vi "Finish.vi"   [LabVIEW 2019]
doc: "This VIcloses device references, sends final commands to the network tables and the joysticks, and terminates all command and control loops."
uses:
  refnums.vi
  <vilib>/Rock Robotics/WPI/Utilities/WPI_GetSetVariantRefNum.vi
types:
  T1 = typedef "WPI_PotentiometerDevRef.ctl" = cluster{"DevStatus":errorcluster, "Analog Channel":T2, "Invert Output":bool}
  T2 = typedef "FPGA_AIChannel.ctl" = enum8{"AI 0", "AI 1", "AI 2", "AI 3", "AI MXP 0", "AI MXP 1", "AI MXP 2", "AI MXP 3", "Invalid"}
  T3 = typedef "WPI_MotorControlDeviceRef.ctl" = cluster{"DeviceStatus":errorcluster, "Type":T4, "PWM":cluster{"PWM Channel":T5, "DeadBand":T6}, "CAN":cluster{"Device Number":u8, "SetOutput VI Ref":variant, "GetOutput VI Ref":variant, "Enable VI Ref":variant, "Disable VI Ref":variant, "Data":variant}, "Invert":bool, "DIO PWM":cluster{"PWM \"Enable\" Channel":T5, "DIOChannel":T7, "PWM Rate":dbl}}
  T4 = typedef "WPI_MotorControlType.ctl" = enum16{"PWM", "CAN", "DIO PWM"}
  T5 = typedef "FPGA_DIOPWMChannel.ctl" = enum8{"PWM 0", "PWM 1", "PWM 2", "PWM 3", "PWM 4", "PWM 5", "PWM 6", "PWM 7", "PWM 8", "PWM 9", "PWM MXP 0", "PWM MXP 1", "PWM MXP 2", "PWM MXP 3", "PWM MXP 4", "PWM MXP 5", "PWM MXP 6", "PWM MXP 7", "PWM MXP 8", "PWM MXP 9", "Invalid"}
  T6 = typedef "WPI_PWMDeadband.ctl" = cluster{"Name":string, "maxPositivePwm":i32, "minPositivePwm":i32, "centerPwm":i32, "maxNegativePwm":i32, "minNegativePwm":i32, "angularRange":u16}
  T7 = typedef "FPGA_DIOChannel.ctl" = enum8{"DIO 0", "DIO 1", "DIO 2", "DIO 3", "DIO 4", "DIO 5", "DIO 6", "DIO 7", "DIO 8", "DIO 9", "DIO MXP 0", "DIO MXP 1", "DIO MXP 2", "DIO MXP 3", "DIO MXP 4", "DIO MXP 5", "DIO MXP 6", "DIO MXP 7", "DIO MXP 8", "DIO MXP 9", "DIO MXP 10", "DIO MXP 11", "DIO MXP 12", "DIO MXP 13", "DIO MXP 14", "DIO MXP 15", "SPI Port CS1", "SPI Port CS2", "SPI Port CS3", "SPI Port MISO", "SPI Port MOSI", "Invalid"}
  T8 = typedef "WPI_SolenoidDevRef.ctl" = cluster{"DevStatus":errorcluster, "Pneumatics Control Module":u8, "Forward Solenoid Channel":T9, "Reverse Solenoid Channel":T9}
  T9 = typedef "WPI_SolenoidChannel.ctl" = enum8{"Solenoid 0", "Solenoid 1", "Solenoid 2", "Solenoid 3", "Solenoid 4", "Solenoid 5", "Solenoid 6", "Solenoid 7", "Invalid"}
  T10 = typedef "WPI_AnalogChannelDevRef.ctl" = cluster{"DevStatus":errorcluster, "Analog Channel":T2}
  T11 = typedef "WPI_CounterDevRef.ctl" = cluster{"DevStatus":errorcluster, "CntIndex":T12}
  T12 = typedef "FPGA_CounterCtrSystemIndex.ctl" = enum8{"Ctr 0", "Ctr 1", "Ctr 2", "Ctr 3", "Ctr 4", "Ctr 5", "Ctr 6", "Ctr 7", "Invalid"}
  T13 = typedef "WPI_JoystickDevRef.ctl" = cluster{"Device":T14}
  T14 = typedef "WPI_JoystickDeviceEnum.ctl" = enum16{"USB 0", "USB 1", "USB 2", "USB 3", "USB 4", "USB 5"}
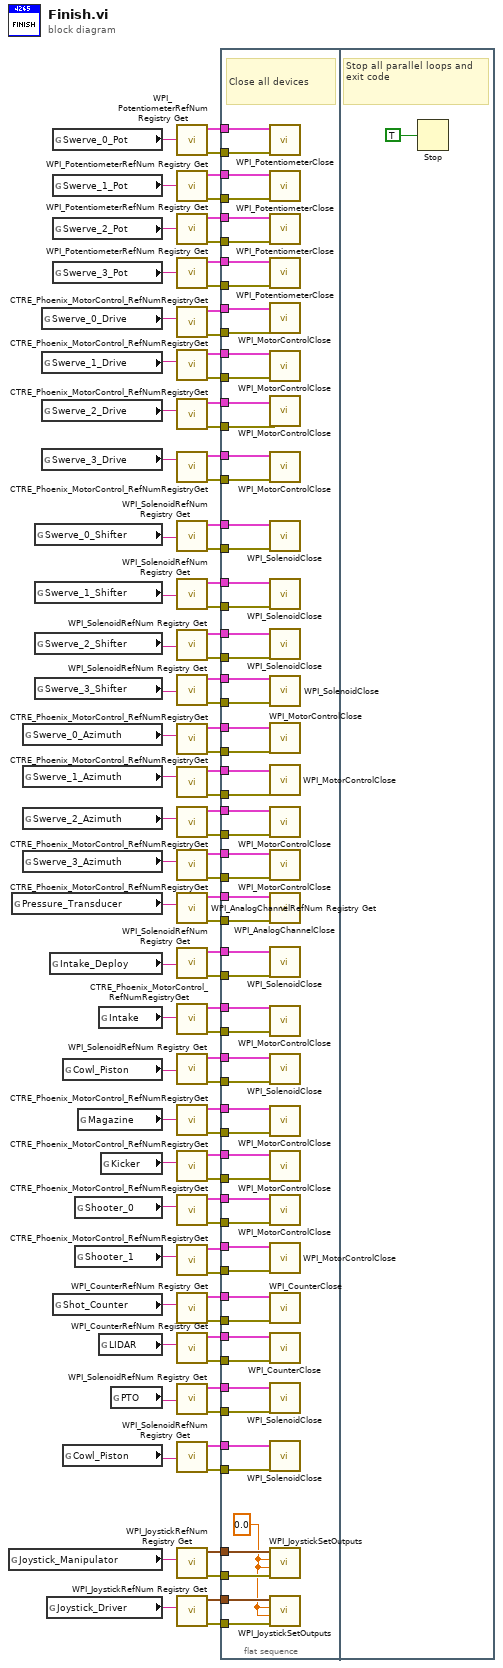
[diagram p0: block diagram]
diagram:
  n1 = global read "refnums.vi" "Joystick_Manipulator"() -> (w72:string)
  n2 = global read "refnums.vi" "Pressure_Transducer"() -> (w78:string)
  n3 = global read "refnums.vi" "Swerve_0_Azimuth"() -> (w48:string)
  n4 = global read "refnums.vi" "Swerve_1_Azimuth"() -> (w47:string)
  n5 = global read "refnums.vi" "Swerve_2_Azimuth"() -> (w46:string)
  n6 = global read "refnums.vi" "Swerve_3_Azimuth"() -> (w45:string)
  n7 = global read "refnums.vi" "Swerve_0_Shifter"() -> (w31:string)
  n8 = global read "refnums.vi" "Swerve_1_Shifter"() -> (w32:string)
  n9 = global read "refnums.vi" "Swerve_2_Shifter"() -> (w33:string)
  n10 = global read "refnums.vi" "Swerve_3_Shifter"() -> (w60:string)
  n11 = global read "refnums.vi" "Swerve_0_Drive"() -> (w57:string)
  n12 = global read "refnums.vi" "Swerve_1_Drive"() -> (w54:string)
  n13 = global read "refnums.vi" "Swerve_2_Drive"() -> (w52:string)
  n14 = global read "refnums.vi" "Swerve_3_Drive"() -> (w63:string)
  n15 = global read "refnums.vi" "Joystick_Driver"() -> (w67:string)
  n16 = global read "refnums.vi" "Intake_Deploy"() -> (w75:string)
  n17 = global read "refnums.vi" "Swerve_0_Pot"() -> (w90:string)
  n18 = global read "refnums.vi" "Swerve_1_Pot"() -> (w88:string)
  n19 = global read "refnums.vi" "Swerve_2_Pot"() -> (w87:string)
  n20 = global read "refnums.vi" "Swerve_3_Pot"() -> (w86:string)
  n21 = global read "refnums.vi" "Shot_Counter"() -> (w24:string)
  n22 = global read "refnums.vi" "Cowl_Piston"() -> (w23:string)
  n23 = global read "refnums.vi" "Cowl_Piston"() -> (w6:string)
  n24 = global read "refnums.vi" "Shooter_0"() -> (w12:string)
  n25 = global read "refnums.vi" "Shooter_1"() -> (w15:string)
  n26 = global read "refnums.vi" "Magazine"() -> (w20:string)
  n27 = global read "refnums.vi" "Intake"() -> (w36:string)
  n28 = global read "refnums.vi" "LIDAR"() -> (w66:string)
  n29 = global read "refnums.vi" "Kicker"() -> (w9:string)
  n30 = global read "refnums.vi" "PTO"() -> (w5:string)
  n31 = call <vilib>:"WPI_PotentiometerRefNum Registry Get.vi"("refnum name"=w90) -> ("error out"=w82:errorcluster, "PotDevRef"=w89:T1)  [unwired: 9 in]
  n32 = call <vilib>:"WPI_PotentiometerRefNum Registry Get.vi"("refnum name"=w88) -> ("error out"=w81:errorcluster, "PotDevRef"=w85:T1)  [unwired: 9 in]
  n33 = call <vilib>:"WPI_PotentiometerRefNum Registry Get.vi"("refnum name"=w87) -> ("error out"=w80:errorcluster, "PotDevRef"=w84:T1)  [unwired: 9 in]
  n34 = call <vilib>:"WPI_PotentiometerRefNum Registry Get.vi"("refnum name"=w86) -> ("error out"=w79:errorcluster, "PotDevRef"=w83:T1)  [unwired: 9 in]
  n35 = call <vilib>:"CTRE_Phoenix_MotorControl_RefNumRegistryGet.vi"("refnum name"=w57) -> ("error out"=w55:errorcluster, "PhoenixMotorControlDevRef"=w56:T3)  [unwired: 9 in]
  n36 = call <vilib>:"CTRE_Phoenix_MotorControl_RefNumRegistryGet.vi"("refnum name"=w54) -> ("error out"=w49:errorcluster, "PhoenixMotorControlDevRef"=w53:T3)  [unwired: 9 in]
  n37 = call <vilib>:"CTRE_Phoenix_MotorControl_RefNumRegistryGet.vi"("refnum name"=w52) -> ("error out"=w50:errorcluster, "PhoenixMotorControlDevRef"=w51:T3)  [unwired: 9 in]
  n38 = call <vilib>:"CTRE_Phoenix_MotorControl_RefNumRegistryGet.vi"("refnum name"=w63) -> ("error out"=w61:errorcluster, "PhoenixMotorControlDevRef"=w62:T3)  [unwired: 9 in]
  n39 = call <vilib>:"WPI_SolenoidRefNum Registry Get.vi"("refnum name"=w31) -> ("error out"=w29:errorcluster, "SolenoidDevRef"=w30:T8)  [unwired: 9 in]
  n40 = call <vilib>:"WPI_SolenoidRefNum Registry Get.vi"("refnum name"=w32) -> ("error out"=w27:errorcluster, "SolenoidDevRef"=w28:T8)  [unwired: 9 in]
  n41 = call <vilib>:"WPI_SolenoidRefNum Registry Get.vi"("refnum name"=w33) -> ("error out"=w25:errorcluster, "SolenoidDevRef"=w26:T8)  [unwired: 9 in]
  n42 = call <vilib>:"WPI_SolenoidRefNum Registry Get.vi"("refnum name"=w60) -> ("error out"=w58:errorcluster, "SolenoidDevRef"=w59:T8)  [unwired: 9 in]
  n43 = call <vilib>:"CTRE_Phoenix_MotorControl_RefNumRegistryGet.vi"("refnum name"=w48) -> ("error out"=w40:errorcluster, "PhoenixMotorControlDevRef"=w44:T3)  [unwired: 9 in]
  n44 = call <vilib>:"CTRE_Phoenix_MotorControl_RefNumRegistryGet.vi"("refnum name"=w47) -> ("error out"=w39:errorcluster, "PhoenixMotorControlDevRef"=w43:T3)  [unwired: 9 in]
  n45 = call <vilib>:"CTRE_Phoenix_MotorControl_RefNumRegistryGet.vi"("refnum name"=w46) -> ("error out"=w38:errorcluster, "PhoenixMotorControlDevRef"=w42:T3)  [unwired: 9 in]
  n46 = call <vilib>:"CTRE_Phoenix_MotorControl_RefNumRegistryGet.vi"("refnum name"=w45) -> ("error out"=w37:errorcluster, "PhoenixMotorControlDevRef"=w41:T3)  [unwired: 9 in]
  n47 = call <vilib>:"WPI_AnalogChannelRefNum Registry Get.vi"("refnum name"=w78) -> ("error out"=w76:errorcluster, "AIDeviceRef"=w77:T10)  [unwired: 9 in]
  n48 = call <vilib>:"WPI_SolenoidRefNum Registry Get.vi"("refnum name"=w75) -> ("error out"=w73:errorcluster, "SolenoidDevRef"=w74:T8)  [unwired: 9 in]
  n49 = call <vilib>:"CTRE_Phoenix_MotorControl_RefNumRegistryGet.vi"("refnum name"=w36) -> ("error out"=w34:errorcluster, "PhoenixMotorControlDevRef"=w35:T3)  [unwired: 9 in]
  n50 = call <vilib>:"WPI_SolenoidRefNum Registry Get.vi"("refnum name"=w23) -> ("error out"=w21:errorcluster, "SolenoidDevRef"=w22:T8)  [unwired: 9 in]
  n51 = call <vilib>:"CTRE_Phoenix_MotorControl_RefNumRegistryGet.vi"("refnum name"=w20) -> ("error out"=w18:errorcluster, "PhoenixMotorControlDevRef"=w19:T3)  [unwired: 9 in]
  n52 = call <vilib>:"CTRE_Phoenix_MotorControl_RefNumRegistryGet.vi"("refnum name"=w9) -> ("error out"=w7:errorcluster, "PhoenixMotorControlDevRef"=w8:T3)  [unwired: 9 in]
  n53 = call <vilib>:"CTRE_Phoenix_MotorControl_RefNumRegistryGet.vi"("refnum name"=w12) -> ("error out"=w10:errorcluster, "PhoenixMotorControlDevRef"=w11:T3)  [unwired: 9 in]
  n54 = call <vilib>:"CTRE_Phoenix_MotorControl_RefNumRegistryGet.vi"("refnum name"=w15) -> ("error out"=w13:errorcluster, "PhoenixMotorControlDevRef"=w14:T3)  [unwired: 9 in]
  n55 = call <vilib>:"WPI_CounterRefNum Registry Get.vi"("refnum name"=w24) -> ("error out"=w16:errorcluster, "CounterDevRef"=w17:T11)  [unwired: 9 in]
  n56 = call <vilib>:"WPI_CounterRefNum Registry Get.vi"("refnum name"=w66) -> ("error out"=w64:errorcluster, "CounterDevRef"=w65:T11)  [unwired: 9 in]
  n57 = call <vilib>:"WPI_SolenoidRefNum Registry Get.vi"("refnum name"=w5) -> ("error out"=w3:errorcluster, "SolenoidDevRef"=w4:T8)  [unwired: 9 in]
  n58 = call <vilib>:"WPI_SolenoidRefNum Registry Get.vi"("refnum name"=w6) -> ("error out"=w1:errorcluster, "SolenoidDevRef"=w2:T8)  [unwired: 9 in]
  n59 = call <vilib>:"WPI_JoystickRefNum Registry Get.vi"("refnum name"=w72) -> ("error out"=w70:errorcluster, "JoystickDevRef"=w71:T13)  [unwired: 9 in]
  n60 = call <vilib>:"WPI_JoystickRefNum Registry Get.vi"("refnum name"=w67) -> ("error out"=w68:errorcluster, "JoystickDevRef"=w69:T13)  [unwired: 9 in]
  n61 = flat-sequence {
    tunnel: w89 -> [w151]
    tunnel: w85 -> [w150]
    tunnel: w84 -> [w149]
    tunnel: w83 -> [w148]
    tunnel: w56 -> [w147]
    tunnel: w53 -> [w146]
    tunnel: w82 -> [w145]
    tunnel: w81 -> [w144]
    tunnel: w80 -> [w143]
    tunnel: w79 -> [w142]
    tunnel: w55 -> [w141]
    tunnel: w77 -> [w140]
    tunnel: w76 -> [w139]
    tunnel: w74 -> [w138]
    tunnel: w73 -> [w137]
    tunnel: w71 -> [w136]
    tunnel: w70 -> [w135]
    tunnel: w69 -> [w134]
    tunnel: w68 -> [w133]
    tunnel: w65 -> [w131]
    tunnel: w64 -> [w130]
    tunnel: w62 -> [w129]
    tunnel: w61 -> [w128]
    tunnel: w59 -> [w127]
    tunnel: w58 -> [w126]
    tunnel: w51 -> [w125]
    tunnel: w50 -> [w124]
    tunnel: w49 -> [w123]
    tunnel: w44 -> [w122]
    tunnel: w43 -> [w121]
    tunnel: w42 -> [w120]
    tunnel: w41 -> [w119]
    tunnel: w40 -> [w118]
    tunnel: w39 -> [w117]
    tunnel: w38 -> [w116]
    tunnel: w37 -> [w115]
    tunnel: w35 -> [w114]
    tunnel: w34 -> [w113]
    tunnel: w30 -> [w112]
    tunnel: w29 -> [w111]
    tunnel: w28 -> [w110]
    tunnel: w27 -> [w109]
    tunnel: w26 -> [w108]
    tunnel: w25 -> [w107]
    tunnel: w22 -> [w106]
    tunnel: w21 -> [w105]
    tunnel: w19 -> [w104]
    tunnel: w18 -> [w103]
    tunnel: w17 -> [w102]
    tunnel: w16 -> [w101]
    tunnel: w13 -> [w100]
    tunnel: w14 -> [w99]
    tunnel: w11 -> [w98]
    tunnel: w10 -> [w97]
    tunnel: w8 -> [w96]
    tunnel: w7 -> [w95]
    tunnel: w4 -> [w94]
    tunnel: w3 -> [w93]
    tunnel: w2 -> [w92]
    tunnel: w1 -> [w91]
    frame #0 {
      w132 = sgl 0.0 ("Left Rumble")
      # "Close all devices"
      n62 = call <vilib>:"WPI_PotentiometerClose.vi"("error in"=w145, "PotDevRef"=w151) -> ()  [unwired: 9 in, 1 out]
      n63 = call <vilib>:"WPI_PotentiometerClose.vi"("error in"=w144, "PotDevRef"=w150) -> ()  [unwired: 9 in, 1 out]
      n64 = call <vilib>:"WPI_PotentiometerClose.vi"("error in"=w143, "PotDevRef"=w149) -> ()  [unwired: 9 in, 1 out]
      n65 = call <vilib>:"WPI_PotentiometerClose.vi"("error in"=w142, "PotDevRef"=w148) -> ()  [unwired: 9 in, 1 out]
      n66 = call <vilib>:"WPI_MotorControlClose.vi"("error in"=w141, "MotorControlDevRef"=w147) -> ()  [unwired: 9 in, 1 out]
      n67 = call <vilib>:"WPI_MotorControlClose.vi"("error in"=w123, "MotorControlDevRef"=w146) -> ()  [unwired: 9 in, 1 out]
      n68 = call <vilib>:"WPI_MotorControlClose.vi"("error in"=w124, "MotorControlDevRef"=w125) -> ()  [unwired: 9 in, 1 out]
      n69 = call <vilib>:"WPI_MotorControlClose.vi"("error in"=w128, "MotorControlDevRef"=w129) -> ()  [unwired: 9 in, 1 out]
      n70 = call <vilib>:"WPI_SolenoidClose.vi"("error in (no error)"=w111, "SolenoidDevRef"=w112) -> ()  [unwired: 9 in, 1 out]
      n71 = call <vilib>:"WPI_SolenoidClose.vi"("error in (no error)"=w109, "SolenoidDevRef"=w110) -> ()  [unwired: 9 in, 1 out]
      n72 = call <vilib>:"WPI_SolenoidClose.vi"("error in (no error)"=w107, "SolenoidDevRef"=w108) -> ()  [unwired: 9 in, 1 out]
      n73 = call <vilib>:"WPI_SolenoidClose.vi"("error in (no error)"=w126, "SolenoidDevRef"=w127) -> ()  [unwired: 9 in, 1 out]
      n74 = call <vilib>:"WPI_MotorControlClose.vi"("error in"=w118, "MotorControlDevRef"=w122) -> ()  [unwired: 9 in, 1 out]
      n75 = call <vilib>:"WPI_MotorControlClose.vi"("error in"=w117, "MotorControlDevRef"=w121) -> ()  [unwired: 9 in, 1 out]
      n76 = call <vilib>:"WPI_MotorControlClose.vi"("error in"=w116, "MotorControlDevRef"=w120) -> ()  [unwired: 9 in, 1 out]
      n77 = call <vilib>:"WPI_MotorControlClose.vi"("error in"=w115, "MotorControlDevRef"=w119) -> ()  [unwired: 9 in, 1 out]
      n78 = call <vilib>:"WPI_AnalogChannelClose.vi"("error in (no error)"=w139, "AIDeviceRef"=w140) -> ()  [unwired: 9 in, 1 out]
      n79 = call <vilib>:"WPI_SolenoidClose.vi"("error in (no error)"=w137, "SolenoidDevRef"=w138) -> ()  [unwired: 9 in, 1 out]
      n80 = call <vilib>:"WPI_MotorControlClose.vi"("error in"=w113, "MotorControlDevRef"=w114) -> ()  [unwired: 9 in, 1 out]
      n81 = call <vilib>:"WPI_SolenoidClose.vi"("error in (no error)"=w105, "SolenoidDevRef"=w106) -> ()  [unwired: 9 in, 1 out]
      n82 = call <vilib>:"WPI_MotorControlClose.vi"("error in"=w103, "MotorControlDevRef"=w104) -> ()  [unwired: 9 in, 1 out]
      n83 = call <vilib>:"WPI_MotorControlClose.vi"("error in"=w95, "MotorControlDevRef"=w96) -> ()  [unwired: 9 in, 1 out]
      n84 = call <vilib>:"WPI_MotorControlClose.vi"("error in"=w97, "MotorControlDevRef"=w98) -> ()  [unwired: 9 in, 1 out]
      n85 = call <vilib>:"WPI_MotorControlClose.vi"("error in"=w100, "MotorControlDevRef"=w99) -> ()  [unwired: 9 in, 1 out]
      n86 = call <vilib>:"WPI_CounterClose.vi"("error in (no error)"=w101, "CounterDevRef"=w102) -> ()  [unwired: 9 in, 1 out]
      n87 = call <vilib>:"WPI_CounterClose.vi"("error in (no error)"=w130, "CounterDevRef"=w131) -> ()  [unwired: 9 in, 1 out]
      n88 = call <vilib>:"WPI_SolenoidClose.vi"("error in (no error)"=w93, "SolenoidDevRef"=w94) -> ()  [unwired: 9 in, 1 out]
      n89 = call <vilib>:"WPI_SolenoidClose.vi"("error in (no error)"=w91, "SolenoidDevRef"=w92) -> ()  [unwired: 9 in, 1 out]
      n90 = call <vilib>:"WPI_JoystickSetOutputs.vi"("error in (no error)"=w135, "Right Rumble"=w132, "Left Rumble"=w132, "JoystickDevRef"=w136) -> ()  [unwired: 6 in, 2 out]
      n91 = call <vilib>:"WPI_JoystickSetOutputs.vi"("error in (no error)"=w133, "Right Rumble"=w132, "Left Rumble"=w132, "JoystickDevRef"=w134) -> ()  [unwired: 6 in, 2 out]
    }
    frame #1 {
      # "Stop all parallel loops and exit code"
      n92 = Stop(stop? (T)=TRUE ("Quit")) -> ()
    }
  }
